vi "3-2 my_LED_step1.vi"() -> ()   [LabVIEW 2014]
doc: "------------------------------------\nAuther: Koji Ohashi\nCopyright (c) 2020 Japan LabVIEW Users Group, Volunteer members.\nThis VI is released under the MIT License.\nhttp://opensource.org/licenses/mit-license.php\n------------------------------------"
panel:
  out "Current(A)":dbl
  in  "Current Limiting Resistor (ƒ¶)":dbl
  in  "Forward Voltage (V)":dbl
  in  "Power-supply voltage (V)":dbl
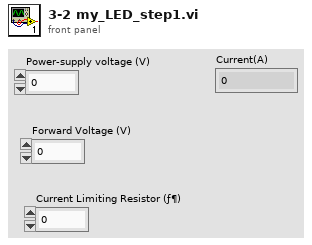
[diagram p1: front panel]
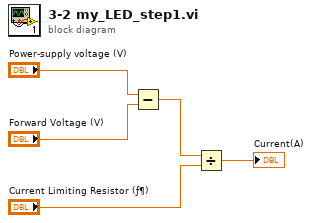
[diagram p0: block diagram]
diagram:
  n1 = Subtract(x="Power-supply voltage (V)", y="Forward Voltage (V)") -> (x-y=w3:dbl)
  n2 = Divide(x=w3, y="Current Limiting Resistor (ƒ¶)") -> (x/y=→"Current(A)":dbl)
